vi "timestamps_functional_global.vi"(5 "Timestamp In":u32, 6 "Buffer Number":i32, 7 "Operation":T1) -> (1 "Last Buffer":i32, 2 "Timestamps":u32[](array[numeric]), 3 "Timestamp Out":u32)   [LabVIEW 2019]
uses:
  TimestampsFunctionalGlobalOperations.ctl
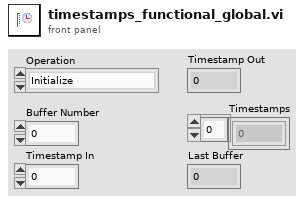
[diagram p1: front panel]
types:
  T1 = typedef "TimestampsFunctionalGlobalOperations.ctl" = enum16{"Initialize", "Dump", "UpdateTime", "ReadTime"}
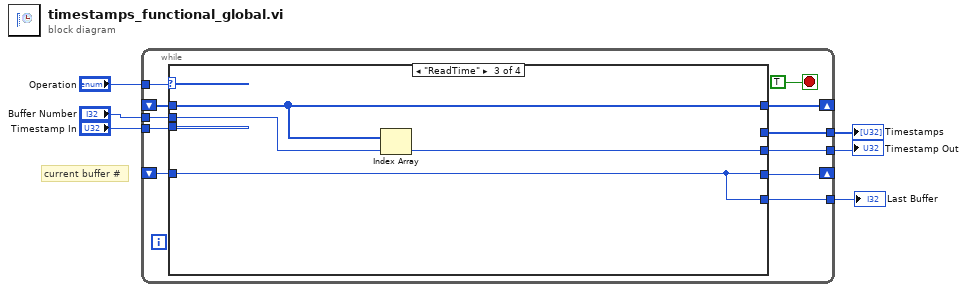
[diagram p0: block diagram]
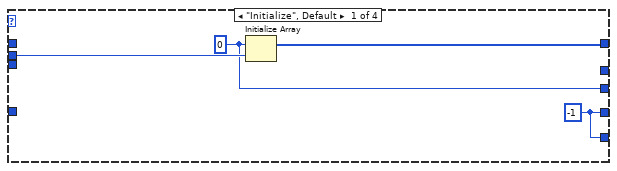
[diagram p2: hidden frame]
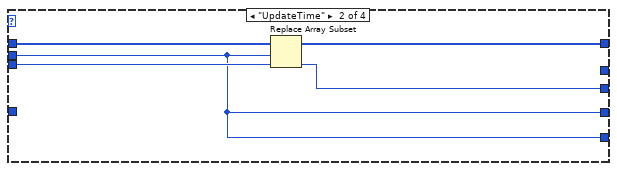
[diagram p3: hidden frame]
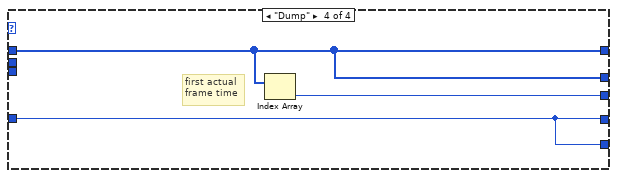
[diagram p4: hidden frame]
diagram:
  # "current buffer #"
  n1 = while {
    shift-right: [w16] -> _
    shift-left: _ -> [w15]
    tunnel: "Timestamp In" -> [w14]
    tunnel: "Operation" -> [w13]
    tunnel: "Buffer Number" -> [w12]
    tunnel: [w11] -> w3
    tunnel: [w10] -> w2
    shift-right: [w9] -> _
    shift-left: _ -> [w8]
    tunnel: [w7] -> w1
    stop <- TRUE stop-if-true
    n2 = case shown="\"ReadTime\"" w13 {
      tunnel: w12 -> [w21 w22 w27 _]
      tunnel: [w20 w24 w28 w31] -> w16
      tunnel: [w19 w23 w29 w32] -> w11
      tunnel: w15 -> [_ w25 w28 w31]
      tunnel: w14 -> [_ w23 _ _]
      tunnel: [_ _ _ w31] -> w10
      tunnel: [w18 w22 w26 w30] -> w9
      tunnel: w8 -> [_ _ w26 w30]
      tunnel: [w18 w22 w26 w30] -> w7
      frame "Initialize", Default {
        w18 = -1 ("Buffer Number")
        w19 = u32 0 ("Buffer Number Out")
        n3 = Initialize Array(w19, w21) -> (w20:u32[])
      }
      frame "UpdateTime" {
        n4 = Replace Array Subset(array=w25, new element=w23, index=w22) -> (w24:u32[])
      }
      frame "ReadTime" {
        n5 = Index Array(array=w28, index=w27) -> (element=w29:u32)
      }
      frame "Dump" {
        # "first actual\nframe time"
        n6 = Index Array(array=w31) -> (element=w32:u32)  [unwired: 1 in]
      }
    }
  }
  "Timestamp Out" <- w3
  "Timestamps" <- w2
  "Last Buffer" <- w1
